vi "retrieveSensorData.vi"(0 "mmHandle in":u64, 1 "path in":path=path "C:/dev/Hexagon-VTD-Custom-Device/Libraries/VC.dll", 5 "packageID":u16, 7 "objIndex":i32, 9 "dataOut":u8[](array[numeric]), 11 "error in (no error)":errorcluster) -> (4 "mmHandle out":u64, 6 "dataOut":u8[](array[numeric]), 15 "error out":errorcluster)   [LabVIEW 2023, in "MM.lvlib"]
uses:
  MM/MM.lvlib
  RDB.lvlib
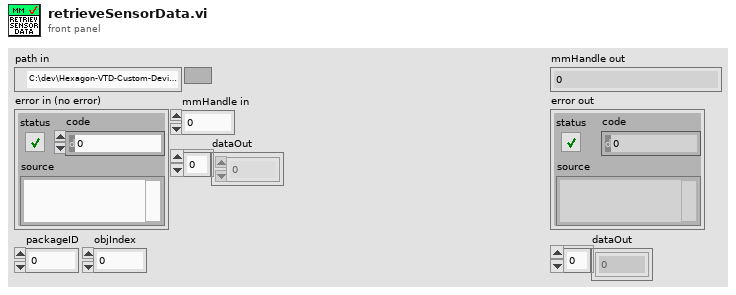
[diagram p1: front panel]
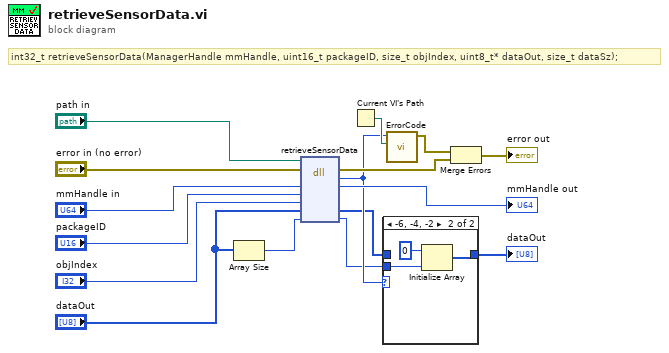
[diagram p0: block diagram]
diagram:
  # "int32_t retrieveSensorData(ManagerHandle mmHandle, uint16_t packageID, size_t objIndex, uint8_t* dataOut, size_t dataSz);"
  n1 = Array Size(array="dataOut") -> (size(s)=w5:i32)
  n2 = dll-call lib="C:/dev/Hexagon-VTD-Custom-Device/Libraries/libMM.dll" fn="retrieveSensorData"(path in="path in", error in="error in (no error)", "paeseHandle"="mmHandle in", "packageID"="packageID", "objIndex"="objIndex", "dataOut"="dataOut", "dataSz"=w5) -> (error out=w12:errorcluster, "return type"=w4:i32, "paeseHandle"=→"mmHandle out":u64, "dataOut"=w3:u8[], "dataSz"=w1:i32)  [unwired: 3 in, 1 out]
  n3 = Current VI's Path() -> (path=w9:path)
  n4 = case shown="-6, -4, -2" w4 {
    tunnel: w3 -> [w17 _]
    tunnel: [w17 w18] -> w2
    tunnel: w1 -> [_ w20]
    frame 0, Default {
    }
    frame -6, -4, -2 {
      n5 = Initialize Array(u8 0, w20) -> (w18:u8[])
    }
  }
  "dataOut" <- w2
  n6 = call "ErrorCode.vi"("parent VI path"=w9, "return type"=w4) -> ("error out"=w13:errorcluster)  [unwired: 9 in]
  n7 = Merge Errors(w13, w12) -> (→"error out":errorcluster)
